vi "Measure.vi"(6 "Channel":i32(ring)=1 items=["Channel 1"=1, "Channel 2"=2, "Channel 3"=3, "Channel 4"=4, "Channel 5"=5, "Channel 6"=6, "Channel 7"=7, "Channel 8"=8, "Channel 8"=9, "Channel 10"=10, "Channel 11"=11, "Channel 12"=12, "Channel 13"=13, "Channel 14"=14, "Channel 15"=15, "Channel 16"=16], 7 "error in":errorcluster, 8 "Max Timeout(ms)":u32=10000, 9 "Measure Type":u16(ring) items=["Current", "Power", "Voltage", "Temperature"], 10 "VISA resource name":refnum<visa-resource-name>) -> (0 "error out":errorcluster, 2 "Measurement":dbl format="%.3g", 3 "VISA resource name out":refnum<visa-resource-name>)   [LabVIEW 2020, in "IT-M3400.lvlib"]
doc: "<b>Measure Type</b>\n0:Current\n1:Power\n2:Voltage\n3:Temperature"
uses:
  IT-M3400.lvlib
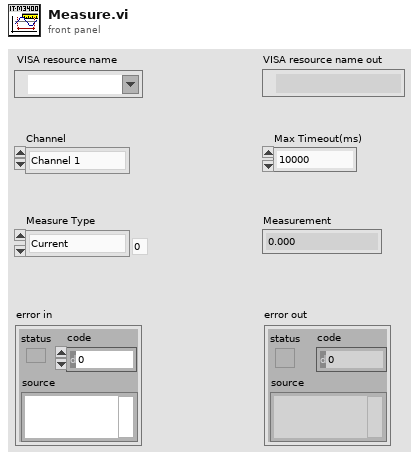
[diagram p1: front panel]
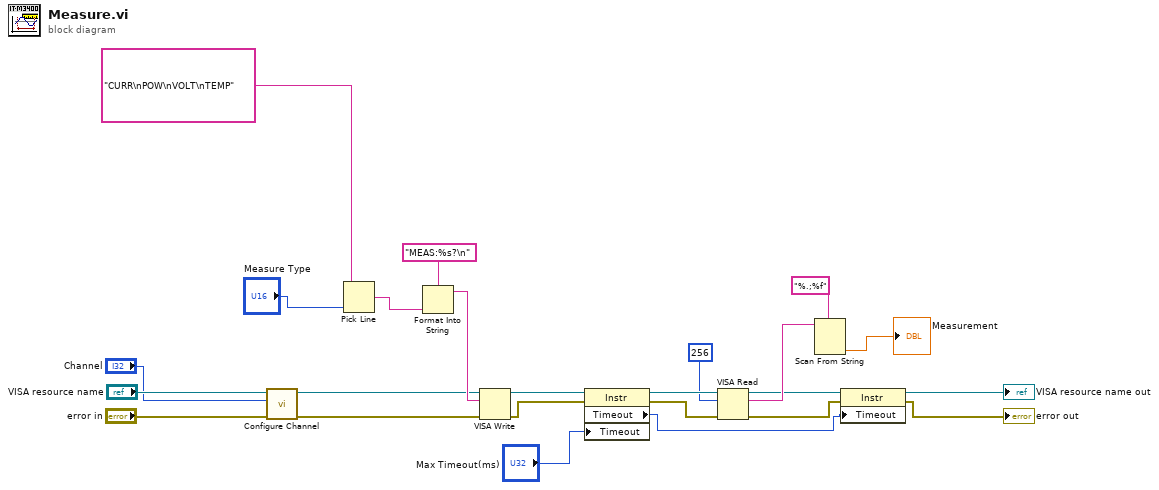
[diagram p0: block diagram]
diagram:
  n1 = call "Configure Channel.vi"("error in"="error in", "Channel"="Channel", "VISA resource name"="VISA resource name") -> ("error out"=w7:errorcluster, "VISA resource name out"=w8:refnum<visa-resource-name>)  [unwired: 7 in]
  n2 = Pick Line(multi-line string="CURR\nPOW\nVOLT\nTEMP", line index="Measure Type") -> (output string=w13:string)  [unwired: 1 in]
  n3 = Format Into String ("格式化写入字符串")(format string="MEAS:%s?\n", w13) -> (resulting string=w23:string)  [unwired: 2 in, 1 out]
  n4 = VISA Write(VISA resource name=w8, write buffer=w23, error in (no error)=w7) -> (VISA resource name out=w11:refnum<visa-resource-name>, error out=w10:errorcluster)  [unwired: 1 out]
  n5 = property class="Instr"(reference=w11, error in=w10, "Timeout"="Max Timeout(ms)") -> (reference out=w20:refnum<visa-resource-name>, error out=w19:errorcluster, "Timeout"=w9:u32)
  n6 = VISA Read(VISA resource name=w20, byte count=256, error in (no error)=w19) -> (VISA resource name out=w16:refnum<visa-resource-name>, read buffer=w22:string, error out=w12:errorcluster)  [unwired: 1 out]
  n7 = Scan From String(format string="%.;%f", input string=w22) -> (output 1=→"Measurement":dbl)  [unwired: 3 in, 3 out]
  n8 = property class="Instr"(reference=w16, error in=w12, "Timeout"=w9) -> (reference out=→"VISA resource name out":refnum<visa-resource-name>, error out=→"error out":errorcluster)
